vi "OpenFileDialog.vi"(8 "错误输入（无错误）":errorcluster, 9 "Multiselect":bool, 10 "Filter":string, 11 "InitialDirectory":path) -> (0 "错误输出":errorcluster, 1 "Multiselect?":bool, 2 "FileNames":path[](array[path]), 3 "FileName":path)   [LabVIEW 2012]
uses:
  System.Windows.Forms
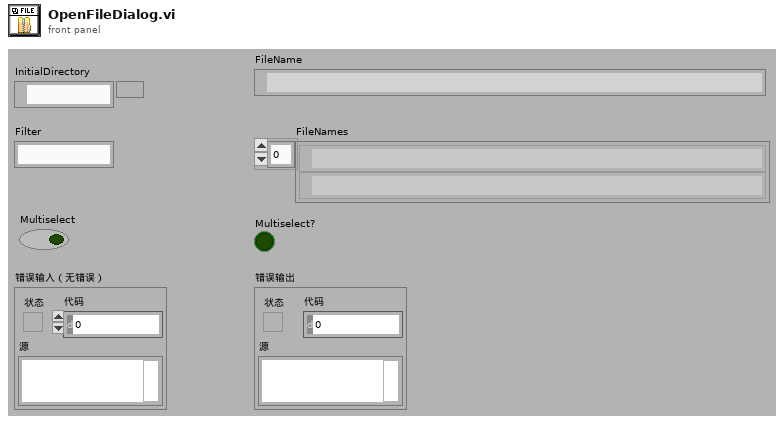
[diagram p1: front panel]
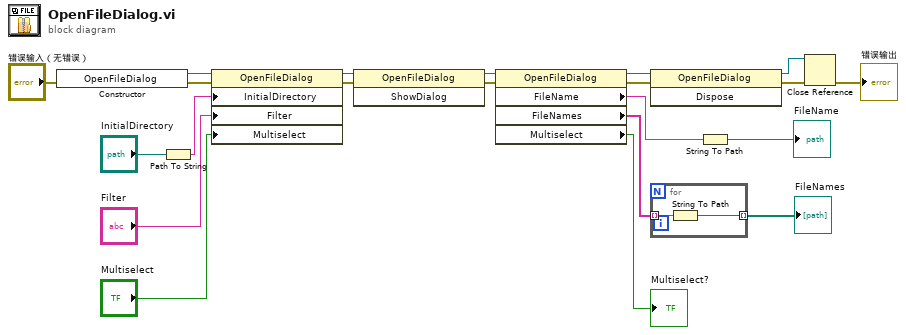
[diagram p0: block diagram]
diagram:
  n1 = constructor class="OpenFileDialog"(error in="错误输入（无错误）") -> (reference out=w21:refnum<k24>, error out=w20:errorcluster)  [unwired: 2 in, 1 out]
  n2 = Path To String(path="InitialDirectory") -> (string=w1:string)
  n3 = property class="OpenFileDialog"(reference=w21, error in=w20, "InitialDirectory"=w1, "Filter"="Filter", "Multiselect"="Multiselect") -> (reference out=w16:refnum<k24>, error out=w15:errorcluster)
  n4 = invoke class="OpenFileDialog" method="ShowDialog"(reference=w16, error in=w15) -> (reference out=w14:refnum<k24>, error out=w13:errorcluster)  [unwired: 1 in, 1 out]
  n5 = property class="OpenFileDialog"(reference=w14, error in=w13) -> (reference out=w11:refnum<k24>, error out=w12:errorcluster, "FileName"=w6:string, "FileNames"=w3:string[], "Multiselect"=→"Multiselect?":bool)
  n6 = invoke class="OpenFileDialog" method="Dispose"(reference=w11, error in=w12) -> (reference out=w10:refnum<k24>, error out=w9:errorcluster)  [unwired: 1 in, 1 out]
  n7 = for {
    tunnel: w3 -> [w23] mode=indexing
    tunnel: [w22] -> w2 mode=indexing
    n8 = String To Path(string=w23) -> (path=w22:path)
  }
  "FileNames" <- w2
  n9 = String To Path(string=w6) -> (path=→"FileName":path)
  n10 = Close Reference(reference=w10, error in (no error)=w9) -> (error out=→"错误输出":errorcluster)
